vi "Get Collision Type.vi"(7 "Combination in":string[](array[string]), 9 "GB Components in":refnum<class "Game Board Component.lvclass">[](array[class]), 11 "Missile in":refnum<class "Missile.lvclass">) -> (2 "Collision out":refnum<class "Collision.lvclass">, 5 "Combination out":string[](array[string]))   [LabVIEW 2021, in "Missile.lvclass"]
doc: "MIT Licence\nCopyright (c) 2024 David Grollier"
uses:
  Missile.lvclass
  Collision/Collision.lvclass
  Game Board Component.lvclass
  Collision/Ball-Edge/Missile-Edge/Missile-Edge.lvclass
  C:/Users/David/Documents/GameSoccerSpace/Source/Collision/Collision.lvclass
  Collision/Ball-Ball/Ball-Missile/Ball-Missile.lvclass
  Collision/Ball-Ball/Missile-Missile/Missile-Missile.lvclass
  Collision/Ball-Goal Post/Missile-Goal Post/Missile-Goal Post.lvclass
  <vilib>/Utility/error.llb/Error Cluster From Error Code.vi
  <vilib>/ErrorRing/Error Ring.xnode
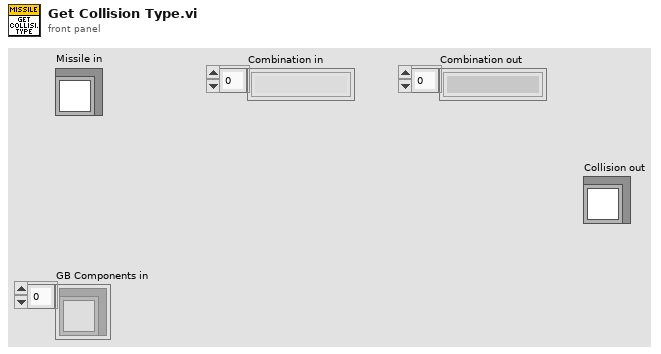
[diagram p1: front panel]
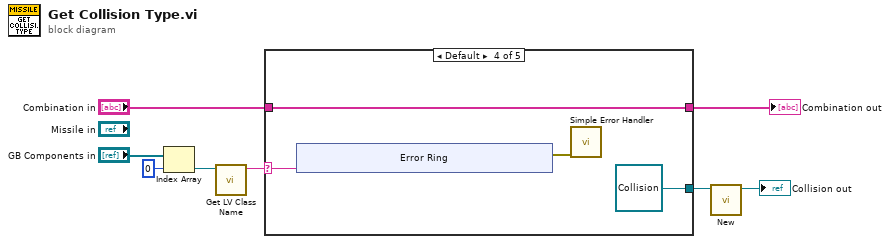
[diagram p0: block diagram]
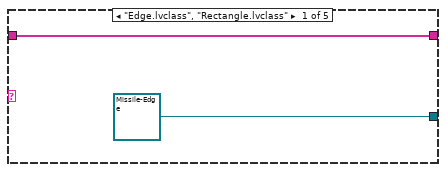
[diagram p2: hidden frame]
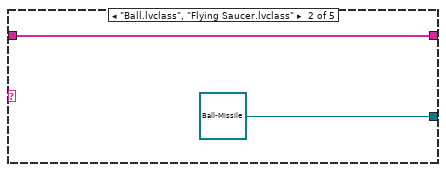
[diagram p3: hidden frame]
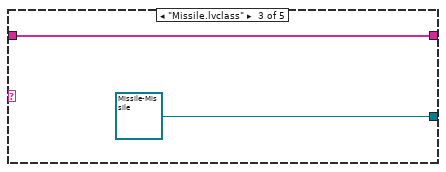
[diagram p4: hidden frame]
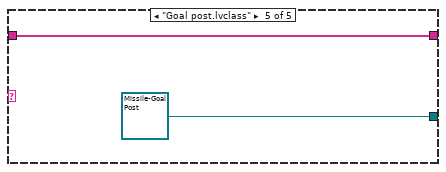
[diagram p5: hidden frame]
diagram:
  n1 = Index Array(array="GB Components in", index=0) -> (element=w5:refnum<class "Game Board Component.lvclass">)
  n2 = call <vilib>:"Get LV Class Name.vi"("object"=w5) -> ("class name"=w4:string)  [unwired: 9 in, 1 out]
  n3 = case shown="Default" w4 {
    selector: w4 -> [_ _ _ w15 _]
    tunnel: [refnum<class "Missile-Edge.lvclass"> refnum ("Missile-Edge.lvclass") refnum<class "Ball-Missile.lvclass"> refnum ("Ball-Missile.lvclass") refnum<class "Missile-Missile.lvclass"> refnum ("Missile-Missile.lvclass") refnum<class "Collision.lvclass"> refnum ("Collision in") refnum<class "Missile-Goal Post.lvclass"> refnum ("Missile-Goal Post.lvclass")] -> w3
    tunnel: "Combination in" -> [w9 w11 w13 w17 w26]
    tunnel: [w9 w11 w13 w17 w26] -> w1
    frame "Edge.lvclass", "Rectangle.lvclass" {
    }
    frame "Ball.lvclass", "Flying Saucer.lvclass" {
    }
    frame "Missile.lvclass" {
    }
    frame Default {
      n4 = xnode "Error Ring"("parameter 0"=w15) -> ("error out"=w16:errorcluster)
      n5 = call <vilib>:"Simple Error Handler.vi"("error in (no error)"=w16) -> ()  [unwired: 4 in, 5 out]
    }
    frame "Goal post.lvclass" {
    }
  }
  "Combination out" <- w1
  n6 = call "New.vi"("Collision in"=w3) -> ("Collision out"=→"Collision out":refnum<class "Collision.lvclass">)  [unwired: 10 in]
